vi "Write.vi"(7 "Message ID (-1)":i32=-1, 8 "error in (no error)":errorcluster, 9 "Device and Axis":string, 10 "Command":string, 11 "VISA resource name":refnum<visa-resource-name>) -> (0 "error out":errorcluster, 3 "VISA resource name out":refnum<visa-resource-name>)   [LabVIEW 2021, in "Zaber A Series.lvlib"]
doc: "Writes a string to the serial port. The communication protocol is detailed at http://www.zaber.com/wiki/Manuals/ASCII_Protocol_Manual. The complete command should be sent to the Command input, but you can optionally input the Device and Axis separately and the VI will bundle these. Additionally the VI will add the required prefix and terminator for the command. \n\nThis VI requires that the Initialize VI has been called with the same serial port."
uses:
  Zaber A Series.lvlib
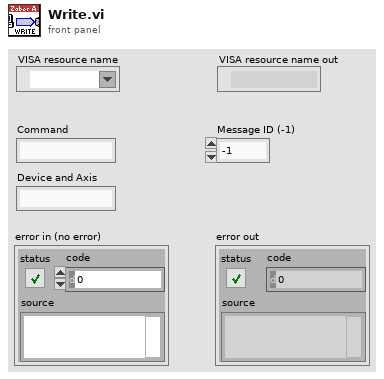
[diagram p1: front panel]
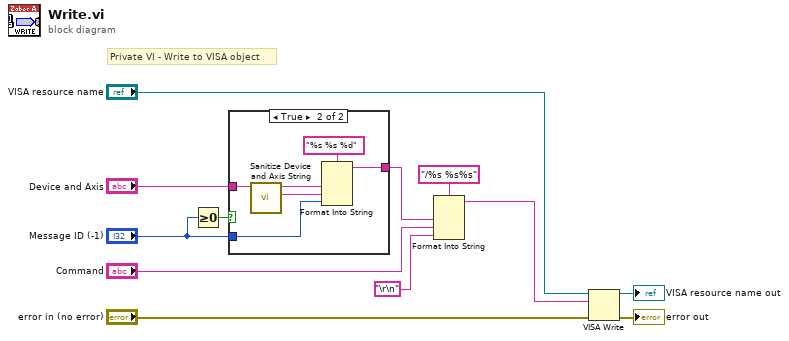
[diagram p0: block diagram]
diagram:
  # "Private VI - Write to VISA object"
  n1 = Greater Or Equal To 0?(x="Message ID (-1)") -> (x >= 0?=w2:bool)
  n2 = case shown="True" w2 {
    tunnel: [w13 w18] -> w6
    tunnel: "Device and Axis" -> [w13 w17]
    tunnel: "Message ID (-1)" -> [_ w14]
    frame False {
    }
    frame True {
      n3 = call "Sanitize Device and Axis String.vi"("Device and Axis"=w17) -> ("Axis Address"=w15:string, "Device Address"=w16:string)  [unwired: 9 in]
      n4 = Format Into String(format string="%s %s %d", w16, w15, w14) -> (resulting string=w18:string)  [unwired: 2 in, 1 out]
    }
  }
  n5 = Format Into String(format string="/%s %s%s", w6, "Command", "\r\n") -> (resulting string=w7:string)  [unwired: 2 in, 1 out]
  n6 = VISA Write(VISA resource name="VISA resource name", write buffer=w7, error in (no error)="error in (no error)") -> (VISA resource name out=→"VISA resource name out":refnum<visa-resource-name>, error out=→"error out":errorcluster)  [unwired: 1 out]
